vi "PIDSetProfile.vi"(0 "Refnum in":refnum<k20>, 1 "Vl":i16, 2 "Vr":i16) -> (8 "PacketOut":u8[](array[numeric]), 9 "error out":errorcluster)   [LabVIEW 2011]
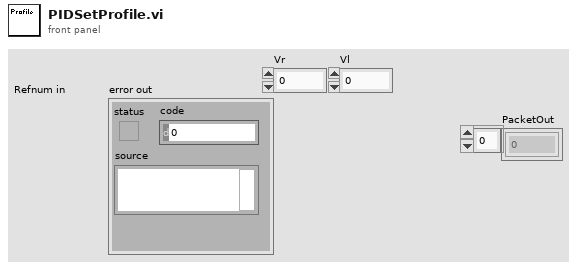
[diagram p1: front panel]
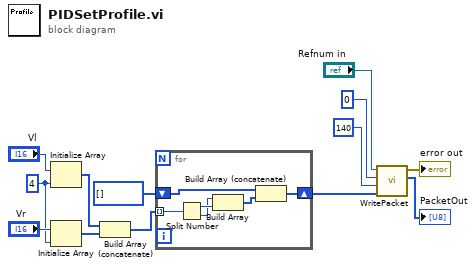
[diagram p0: block diagram]
diagram:
  w7 = 4 ("dimension size")
  n1 = Initialize Array("Vl", w7) -> (w2:i16[])
  n2 = Initialize Array("Vr", w7) -> (w1:i16[])
  n3 = Build Array (concatenate)(w2, w1) -> (w6:i16[])
  n4 = for {
    tunnel: w6 -> [w19] mode=indexing
    shift-right: [w16] -> w4
    shift-left: u8[] [] ("appended array") -> [w18]
    n5 = Split Number(x=w19) -> (hi(x)=w15:u8, lo(x)=w14:u8)
    n6 = Build Array(w14, w15) -> (w17:u8[])
    n7 = Build Array (concatenate)(w18, w17) -> (w16:u8[])
  }
  n8 = call "WritePacket.vi"("Payload"=w4, "Type"=u8 140, "Status"=u8 0, "Refnum in"="Refnum in") -> ("PacketOut"=→"PacketOut":u8[], "error out"=→"error out":errorcluster)  [unwired: 6 in]
